vi "Build Paths.vi"(11 "lvproj Path":path) -> (3 "SET ProjFile Path":path)   [LabVIEW 2013, in "SET Project Data.lvlib"]
doc: "Build Paths.vi\n\nBuild SETProject file path from lvproj path."
uses:
  SET Project Data.lvlib
panel:
  # "Build Paths.vi\n\nBuild SETProject file path from lvproj path"
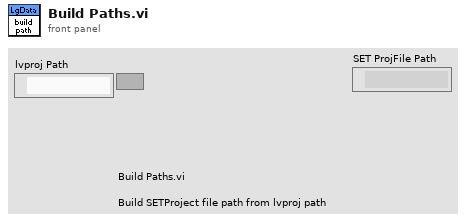
[diagram p1: front panel]
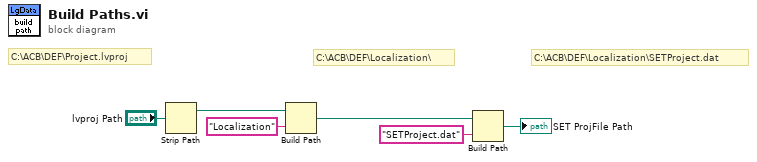
[diagram p0: block diagram]
diagram:
  # "C:\\ACB\\DEF\\Localization\\SETProject.dat"
  # "C:\\ACB\\DEF\\Localization\\"
  # "C:\\ACB\\DEF\\Project.lvproj"
  n1 = Strip Path(path="lvproj Path") -> (stripped path=w4:path)  [unwired: 1 out]
  n2 = Build Path(base path=w4, name or relative path="Localization") -> (appended path=w1:path)
  n3 = Build Path(base path=w1, name or relative path="SETProject.dat") -> (appended path=→"SET ProjFile Path":path)
